vi "run.add_data.vi"(6 "seriesTags":map{string, string}(c390), 8 "error in":errorcluster, 9 "Data Source":T1, 10 "runRid":string, 11 "Nominal Client in":refnum<class "Nominal Client.lvclass">) -> (0 "error out":errorcluster, 2 "Run":refnum<class "Run.lvclass">, 3 "Nominal Client out":refnum<class "Nominal Client.lvclass">, 4 "Full Response":string)   [LabVIEW 2020]
doc: "Adds datasources to the run in question.\n\nThrows if any of the ref names conflict with existing data sources or each other."
uses:
  Nominal Client.lvclass
  Run/Run.lvclass
  290970bd-cfd7-4292-ac98-a7d2a30fd891.vi
  b3265f00-b8ce-49d1-8520-d9de14d3fc6c.vi
  5e51f403-c7b4-4e16-af1a-4d99de4501f8.vi
  20b7332c-9742-4a91-9d1b-dd841378a60a.vi
  1d554ba0-2ab1-45da-9502-233d61096701.vi
  <vilib>/JDP Science/JSONtext/Variant to JSON Text.vi
  <vilib>/JDP Science/JSONtext/Array of Variants to JSON Object.vi
  <vilib>/JDP Science/JSONtext/Set Item.vi
  <vilib>/JDP Science/JSONtext/support/Format JSON Object.vi
  <vilib>/JDP Science/JSONtext/LVClass Serializer/JSONtext LVClass Serializer.lvclass
  Nominal Client.lvclass/Nominal Client.ctl
  <vilib>/JDP Science/JSONtext/JSONtext.lvlib
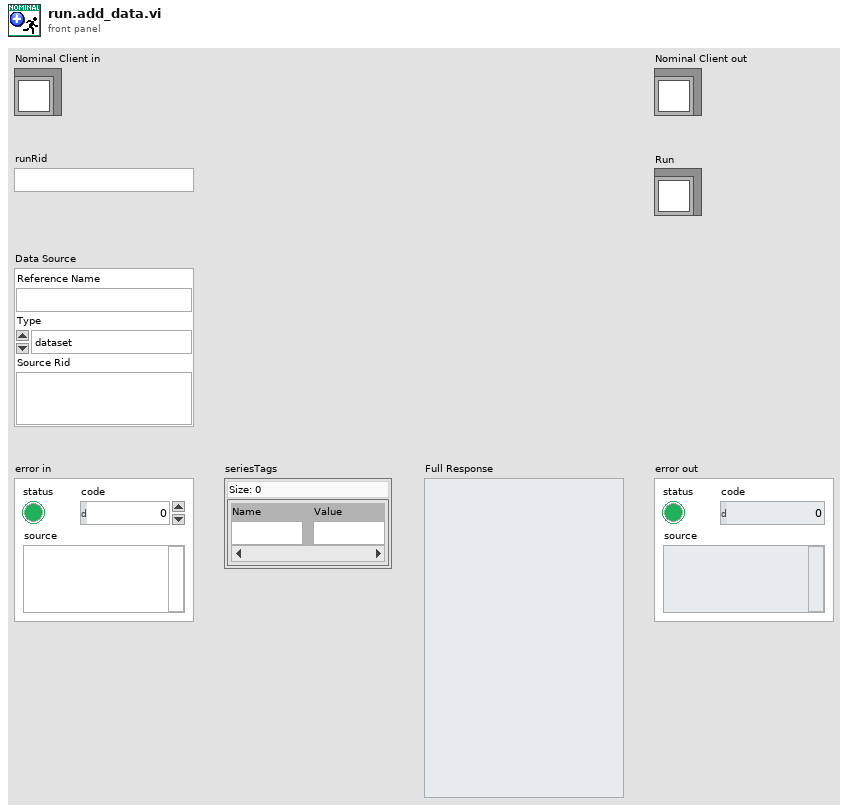
[diagram p1: front panel]
types:
  T1 = cluster{"Reference Name":string, "Type":enum16{"dataset", "connection", "logSet", "video"}, "Source Rid":string}
  T2 = enum16{"dataset", "connection", "logSet", "video"}
  T3 = cluster{"dataSource":cluster{"type":string, "connection":string}, "seriesTags":string}
  T4 = cluster{"dataSource":cluster{"type":string, "logSet":string}, "seriesTags":string}
  T5 = cluster{"dataSource":cluster{"type":string, "video":string}, "seriesTags":string}
  T6 = cluster{"dataSource":cluster{"type":string, "dataset":string}, "seriesTags":string}
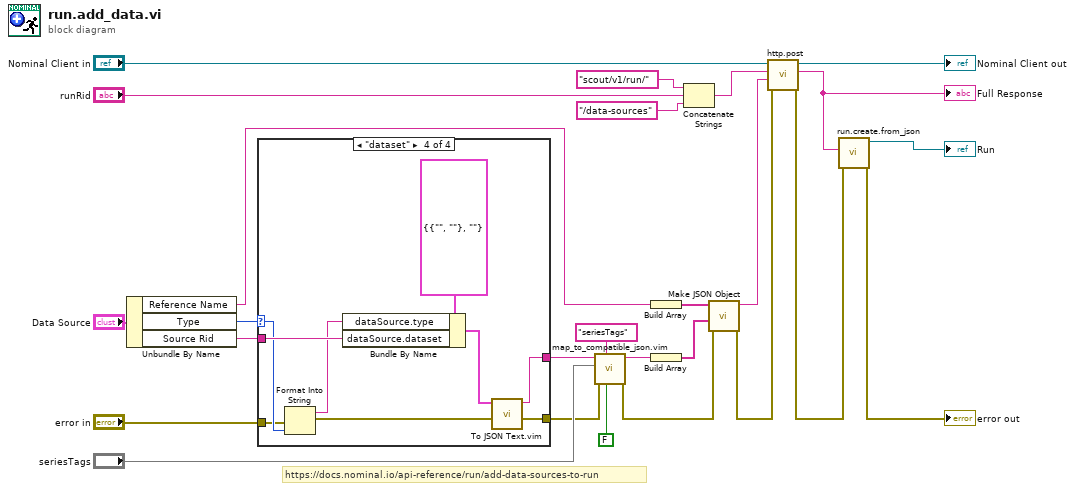
[diagram p0: block diagram]
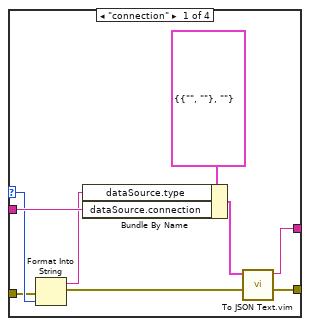
[diagram p2: hidden frame]
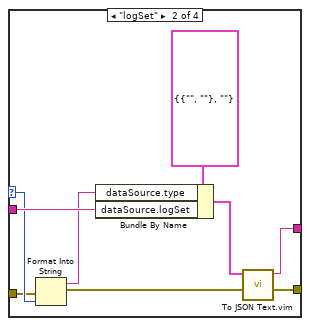
[diagram p3: hidden frame]
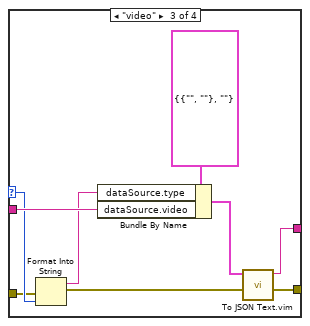
[diagram p4: hidden frame]
diagram:
  # "https://docs.nominal.io/api-reference/run/add-data-sources-to-run"
  n1 = Unbundle By Name("Data Source") -> ("Reference Name"=w5:string, "Type"=w15:T2, "Source Rid"=w16:string)
  n2 = case shown="\"dataset\"" w15 {
    selector: w15 -> [w33 w42 w51 w60]
    tunnel: w16 -> [w34 w43 w52 w61]
    tunnel: [w30 w39 w48 w57] -> w14
    tunnel: [w29 w38 w47 w56] -> w13
    tunnel: "error in" -> [w27 w36 w45 w54]
    frame "connection" {
      n3 = Format Into String(error in=w27, w33) -> (resulting string=w32:string, error out=w28:errorcluster)  [unwired: 2 in]
      n4 = Bundle By Name(cluster=T3 {"dataSource"={"type"="", "connection"=""}, "seriesTags"=""}, "dataSource.type"=w32, "dataSource.connection"=w34) -> (w31:T3)
      n5 = call "To JSON Text.vim"("error in (no error)"=w28, "Anything"=w31) -> ("error out"=w29:errorcluster, "<JSON>"=w30:string)  [unwired: 8 in]
    }
    frame "logSet" {
      n6 = Format Into String(error in=w36, w42) -> (resulting string=w41:string, error out=w37:errorcluster)  [unwired: 2 in]
      n7 = Bundle By Name(cluster=T4 {"dataSource"={"type"="", "logSet"=""}, "seriesTags"=""}, "dataSource.type"=w41, "dataSource.logSet"=w43) -> (w40:T4)
      n8 = call "To JSON Text.vim"("error in (no error)"=w37, "Anything"=w40) -> ("error out"=w38:errorcluster, "<JSON>"=w39:string)  [unwired: 8 in]
    }
    frame "video" {
      n9 = Format Into String(error in=w45, w51) -> (resulting string=w50:string, error out=w46:errorcluster)  [unwired: 2 in]
      n10 = Bundle By Name(cluster=T5 {"dataSource"={"type"="", "video"=""}, "seriesTags"=""}, "dataSource.type"=w50, "dataSource.video"=w52) -> (w49:T5)
      n11 = call "To JSON Text.vim"("error in (no error)"=w46, "Anything"=w49) -> ("error out"=w47:errorcluster, "<JSON>"=w48:string)  [unwired: 8 in]
    }
    frame "dataset" {
      n12 = Format Into String(error in=w54, w60) -> (resulting string=w59:string, error out=w55:errorcluster)  [unwired: 2 in]
      n13 = Bundle By Name(cluster=T6 {"dataSource"={"type"="", "dataset"=""}, "seriesTags"=""}, "dataSource.type"=w59, "dataSource.dataset"=w61) -> (w58:T6)
      n14 = call "To JSON Text.vim"("error in (no error)"=w55, "Anything"=w58) -> ("error out"=w56:errorcluster, "<JSON>"=w57:string)  [unwired: 8 in]
    }
  }
  n15 = call "map_to_compatible_json.vim"("Pretty Print?"=FALSE, "JSON Path"="seriesTags" ("Data Name"), "error in"=w13, "Map"="seriesTags", "JSON in"=w14) -> ("error out"=w8:errorcluster, "JSON out"=w10:string)  [unwired: 5 in]
  n16 = Build Array(w5) -> (w11:string[])
  n17 = Build Array(w10) -> (w9:string[])
  n18 = Concatenate Strings("scout/v1/run/", "runRid", "/data-sources") -> (w21:string)
  n19 = call <vilib>:"Make JSON Object.vi"("error in (no error)"=w8, "JSON Items"=w9, "Item Names"=w11) -> ("error out"=w7:errorcluster, "<JSON>"=w6:string)  [unwired: 7 in]
  n20 = call "http.post.vi"("error in"=w7, "Request body"=w6, "Path"=w21, "Nominal Client in"="Nominal Client in") -> ("error out"=w2:errorcluster, "Response"=w4:string, "Nominal Client out"=→"Nominal Client out":refnum<class "Nominal Client.lvclass">)  [unwired: 4 in, 1 out]
  "Full Response" <- w4
  n21 = call "run.create.from_json.vi"("error in"=w2, "JSON"=w4) -> ("error out"=→"error out":errorcluster, "Run out"=→"Run":refnum<class "Run.lvclass">)  [unwired: 8 in]
